vi "BASE_Reporting.vi"(8 "error in (no error)":errorcluster) -> (0 "error out":errorcluster)   [LabVIEW 2017]
uses:
  <vilib>/addons/database/Connection.llb/DB Tools Open Connec (Path).vi
  <vilib>/Utility/file.llb/Write Delimited Spreadsheet (string).vi
  <vilib>/addons/database/NI_Database_API.lvlib
panel:
  in  "SELECT FILTER":string(combo)="PART_NO"
  in  "Export to Excel":bool
  out "DESCRIPTION":string
  out "Data History Table":string[][](table)
  in  "TO DATE":timestamp
  in  "FROM DATE":timestamp
  in  "Back":bool
  in  "Show Report":bool
  # "BARCODE VERIFICATION SYSTEM REPORTS"
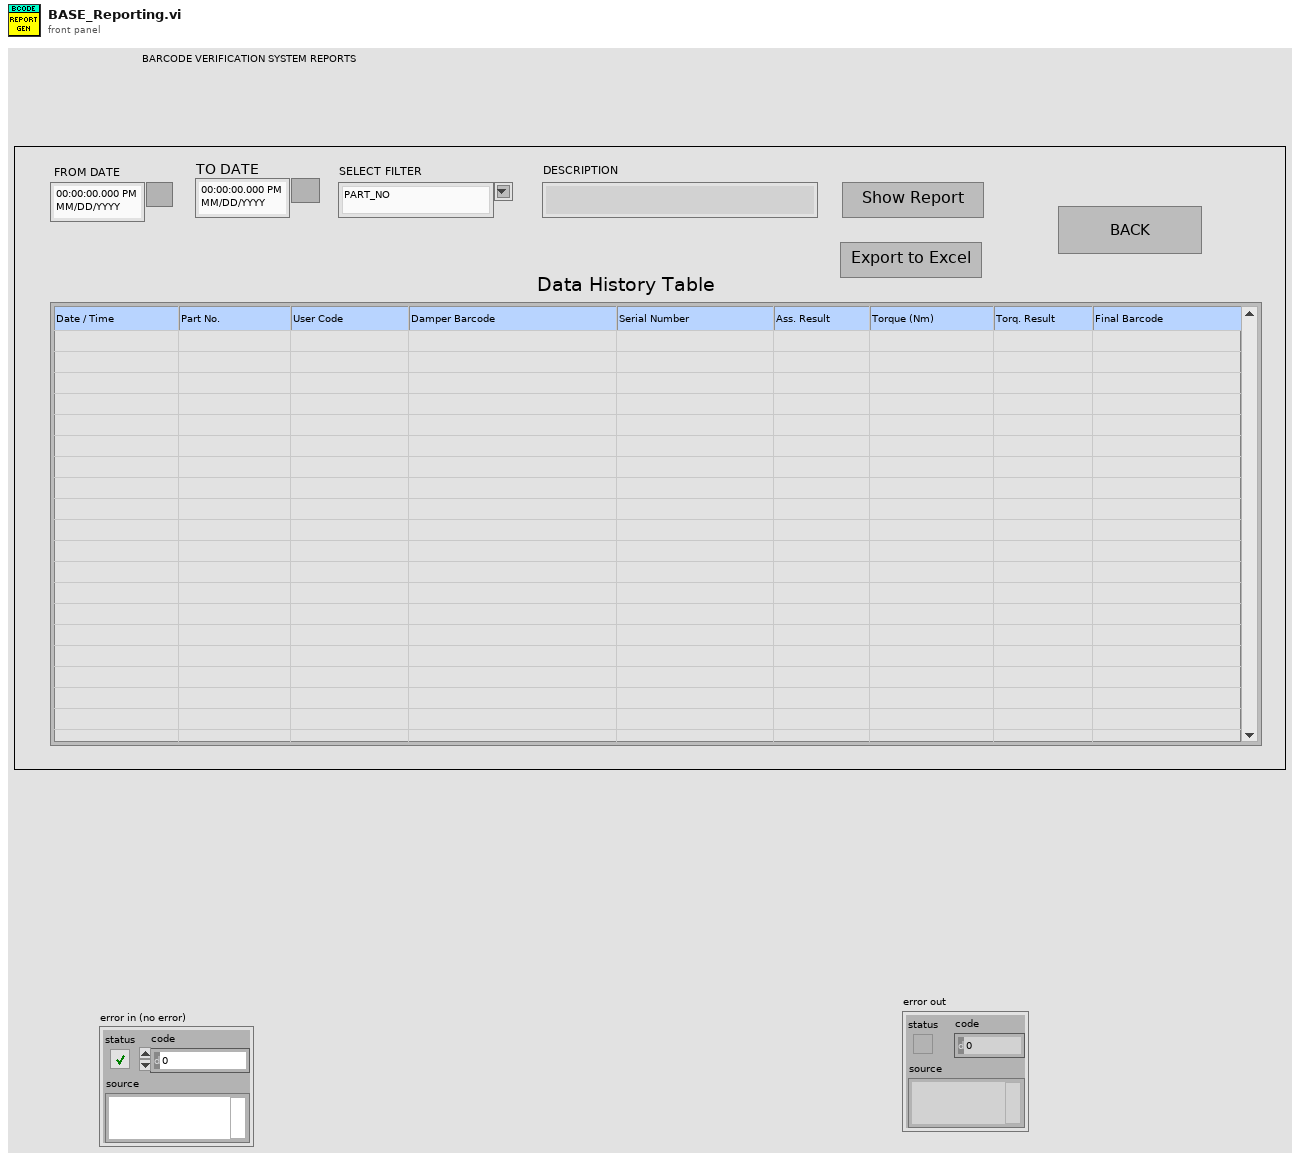
[diagram p1: front panel]
types:
  T1 = enum32{"invalid app kind", "Development System", "Run Time System", "Student Edition", "Embedded LabVIEW", "Evaluation", "Custom"}
  T2 = typedef "NI_Database_API.lvlib/Conn ObjectReference.ctl" = refnum<k1>
  T3 = typedef "LVRowAndColumnTypeDef.ctl" = cluster{"Row":i32, "Column":i32}
  T4 = enum32{"Invalid", "Standard", "Closed", "Hidden", "Minimized", "Maximized"}
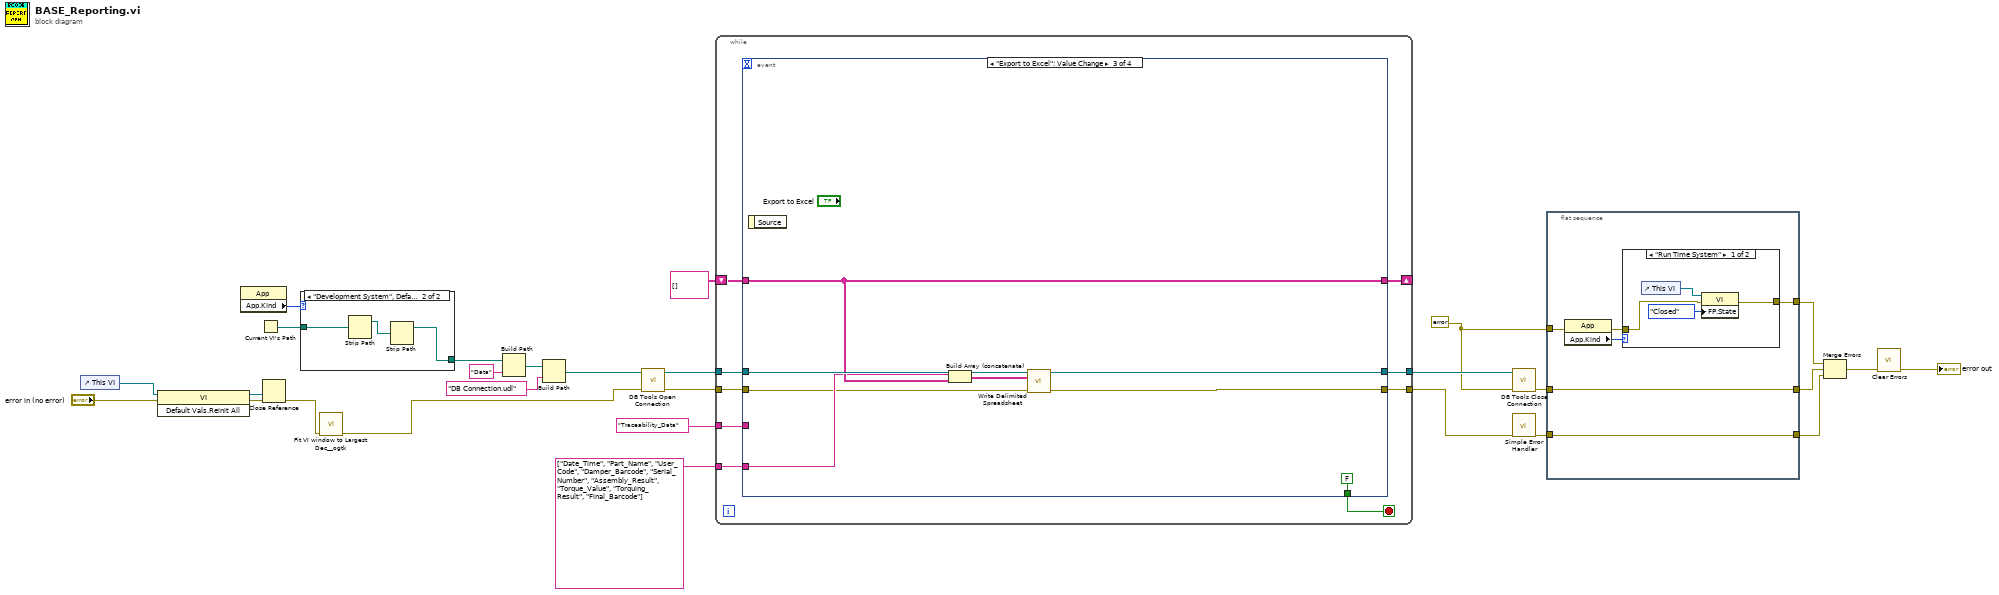
[diagram p0: block diagram]
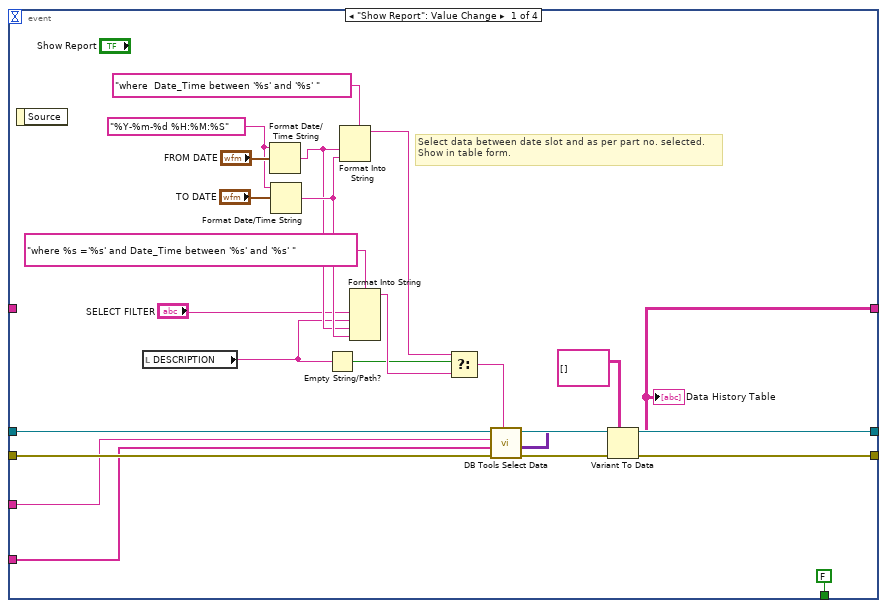
[diagram p3: hidden frame]
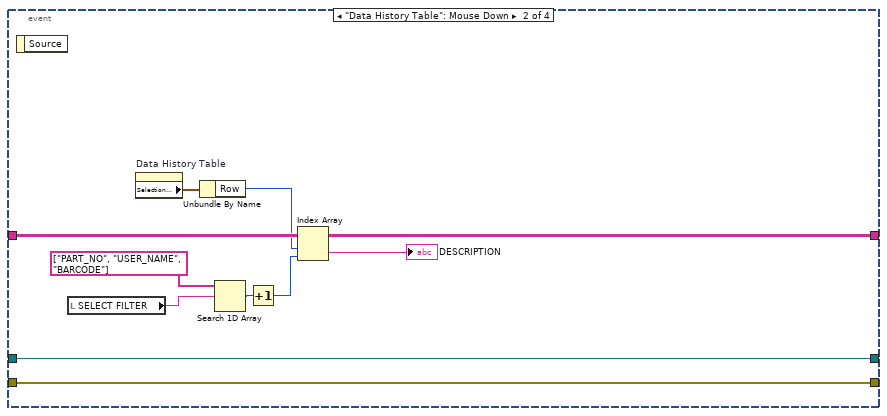
[diagram p4: hidden frame]
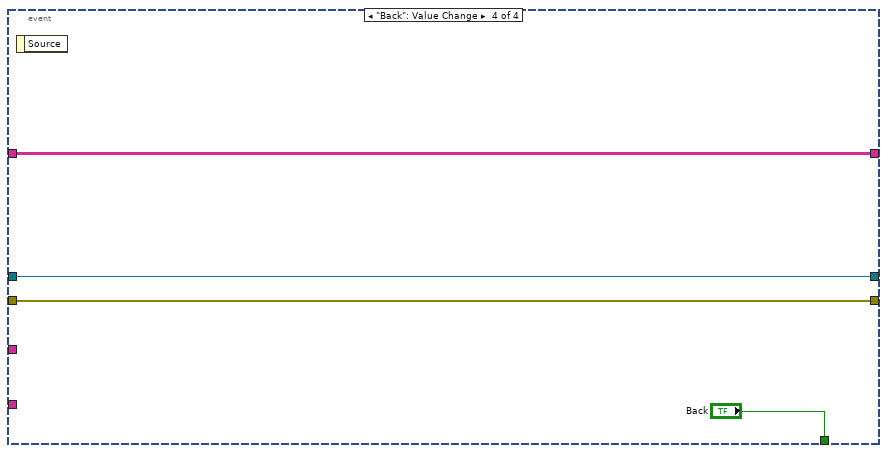
[diagram p5: hidden frame]
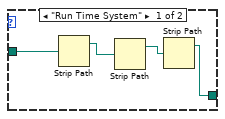
[diagram p6: hidden frame]
diagram:
  w14 = errorcluster {"status"=FALSE, "code"=0, "source"=""} ("error in (no error)")
  n1 = control-ref of="This VI"() -> (w8:refnum<vi>)
  n2 = invoke class="VI" method="Default Vals.Reinit All"(reference=w8, error in="error in (no error)") -> (reference out=w6:refnum<vi>, error out=w5:errorcluster)  [unwired: 1 in, 1 out]
  n3 = property class="App"() -> ("App.Kind"=w24:T1)  [unwired: 2 in, 2 out]
  n4 = Current VI's Path() -> (path=w25:path)
  n5 = Close Reference(reference=w6, error in (no error)=w5) -> (error out=w2:errorcluster)
  n6 = case shown="\"Development System\", Default" w24 {
    tunnel: w25 -> [w30 w34]
    tunnel: [w29 w33] -> w22
    frame "Run Time System" {
      n7 = Strip Path(path=w30) -> (stripped path=w32:path)  [unwired: 1 out]
      n8 = Strip Path(path=w32) -> (stripped path=w31:path)  [unwired: 1 out]
      n9 = Strip Path(path=w31) -> (stripped path=w29:path)  [unwired: 1 out]
    }
    frame "Development System", Default {
      n10 = Strip Path(path=w34) -> (stripped path=w35:path)  [unwired: 1 out]
      n11 = Strip Path(path=w35) -> (stripped path=w33:path)  [unwired: 1 out]
    }
  }
  n12 = call <userlib>:"Fit VI window to Largest Dec__ogtk.vi"("error in (no error)"=w2) -> ("error out"=w1:errorcluster)  [unwired: 5 in, 1 out]
  n13 = Build Path(base path=w22, name or relative path="Data") -> (appended path=w23:path)
  n14 = Build Path(base path=w23, name or relative path="DB Connection.udl") -> (appended path=w19:path)
  n15 = call-poly <vilib>:"DB Tools Open Connection.vi"("error in (no error)"=w1, "connection information"=w19) -> ("error out"=w27:errorcluster, "connection reference"=w28:T2)  [unwired: 6 in]
  n16 = while {
    tunnel: string[] ["Date_Time", "Part_Name", "User_Code", "Damper_Barcode", "Serial_Number", "Assembly_Result", "Torque_Value", "Torquing_Result", "Final_Barcode"] -> [w40]
    tunnel: "Traceability_Data" ("table") -> [w39]
    tunnel: w28 -> [w44]
    tunnel: [w41] -> w26
    tunnel: w27 -> [w43]
    tunnel: [w42] -> w17
    shift-right: [w37] -> _
    shift-left: string[][] [] -> [w36]
    stop <- w38 stop-if-true
    n17 = event shown="[2] \"Export to Excel\": Value Change" {
      selector: _ -> [_ _ _ _]
      dyn-events: _ -> [_ _ _ _]
      timeout: _ -> [_ _ _ _]
      tunnel: w44 -> [w68 w75 w85 w88]
      tunnel: w43 -> [w67 w74 w80 w87]
      tunnel: [w59 w74 w79 w87] -> w42
      tunnel: [w66 w75 w85 w88] -> w41
      tunnel: w40 -> [w65 _ w81 _]
      tunnel: w39 -> [w64 _ _ _]
      tunnel: [FALSE ("Back") _ FALSE ("Back") "Back"] -> w38
      tunnel: [w49 w78 w82 w86] -> w37
      tunnel: w36 -> [_ w78 w82 w86]
      event "Show Report": Value Change {
        w52 = "%Y-%m-%d %H:%M:%S"
        # "Select data between date slot and as per part no. selected.\nShow in table form."
        n18 = event-data() -> ()  [unwired: 1 in, 1 out]
        n19 = local read "DESCRIPTION"() -> (w45:string)
        n20 = Format Date/Time String(time format string (%c)=w52, seconds (now)="FROM DATE") -> (date/time string=w47:string)  [unwired: 1 in]
        n21 = Format Date/Time String(time format string (%c)=w52, seconds (now)="TO DATE") -> (date/time string=w48:string)  [unwired: 1 in]
        n22 = Empty String/Path?(string/path=w45) -> (empty?=w50:bool)
        n23 = Format Into String(format string="where  Date_Time between '%s' and '%s' ", w47, w48) -> (resulting string=w57:string)  [unwired: 2 in, 1 out]
        n24 = Format Into String(format string="where %s ='%s' and Date_Time between '%s' and '%s' ", "SELECT FILTER", w45, w47, w48) -> (resulting string=w58:string)  [unwired: 2 in, 1 out]
        n25 = Select(t=w57, s=w50, f=w58) -> (s? t:f=w51:string)
        n26 = call <vilib>:"DB Tools Select Data.vi"("condition"=w51, "error in (no error)"=w67, "columns"=w65, "table"=w64, "connection reference"=w68) -> ("error out"=w60:errorcluster, "data"=w63:variant[][], "connection reference out"=w66:T2)  [unwired: 1 in]
        n27 = Variant To Data(error in=w60, type=string[][] [], Variant=w63) -> (data=w49:string[][], error out=w59:errorcluster)
        "Data History Table" <- w49
      }
      event "Data History Table": Mouse Down {
        n28 = event-data() -> ()  [unwired: 1 in, 1 out]
        n29 = local read "SELECT FILTER"() -> (w71:string)
        n30 = property on="Data History Table" class="Tbl (strict)"() -> ("Selection Start"=w77:T3)  [unwired: 2 in, 2 out]
        n31 = Unbundle By Name(w77) -> ("Row"=w76:i32)
        n32 = Search 1D Array(1D array=string[] ["PART_NO", "USER_NAME", "BARCODE"], element=w71) -> (index of element=w70:i32)  [unwired: 1 in]
        n33 = Increment(x=w70) -> (x+1=w69:i32)
        n34 = Index Array(array=w78, index (row)=w76, index (col)=w69) -> (element=→"DESCRIPTION":string)
      }
      event "Export to Excel": Value Change {
        n35 = event-data() -> ()  [unwired: 1 in, 1 out]
        n36 = Build Array (concatenate)(w81, w82) -> (w83:string[][])
        n37 = call-poly <vilib>:"Write Delimited Spreadsheet.vi"("2D data"=w83, "error in (no error)"=w80) -> ("error out"=w79:errorcluster)  [unwired: 12 in, 1 out]
      }
      event "Back": Value Change {
        n38 = event-data() -> ()  [unwired: 1 in, 1 out]
      }
    }
  }
  n39 = call <vilib>:"DB Tools Close Connection.vi"("error in (no error)"=w14, "connection reference"=w26) -> ("error out"=w12:errorcluster)  [unwired: 5 in]
  n40 = call <vilib>:"Simple Error Handler.vi"("error in (no error)"=w17) -> ("error out"=w10:errorcluster)  [unwired: 4 in, 4 out]
  n41 = flat-sequence {
    tunnel: [w93] -> w15
    tunnel: w14 -> [w92]
    tunnel: [w91] -> w13
    tunnel: w12 -> [w91]
    tunnel: [w90] -> w11
    tunnel: w10 -> [w90]
    frame #0 {
      n42 = property class="App"(error in=w92) -> (error out=w94:errorcluster, "App.Kind"=w95:T1)  [unwired: 1 in, 1 out]
      n43 = case shown="\"Run Time System\"" w95 {
        tunnel: w94 -> [w97 w100]
        tunnel: [w96 w100] -> w93
        frame "Run Time System" {
          n44 = control-ref of="This VI"() -> (w99:refnum<vi>)
          n45 = property class="VI"(reference=w99, error in=w97, "FP.State"=T4."Closed" ("Front Panel Window:State")) -> (error out=w96:errorcluster)  [unwired: 1 out]
        }
        frame "Development System", Default {
        }
      }
    }
  }
  n46 = Merge Errors(w15, w13, w11) -> (w16:errorcluster)
  n47 = call <vilib>:"Clear Errors.vi"("error in (no error)"=w16) -> ("error out"=→"error out":errorcluster)  [unwired: 5 in, 1 out]
